vi "Get Column Info.vi"(8 "error in (no error)":errorcluster, 9 "Column Name Array":string[](array[string]), 10 "Table Name":string, 11 "Database in":refnum<class "Database.lvclass">) -> (0 "error out":errorcluster, 2 "Column Information Array":T1(array[cluster]), 3 "Database out":refnum<class "Database.lvclass">)   [LabVIEW 2020, in "Database.lvlib" / "Database.lvclass"]
uses:
  Database.lvclass
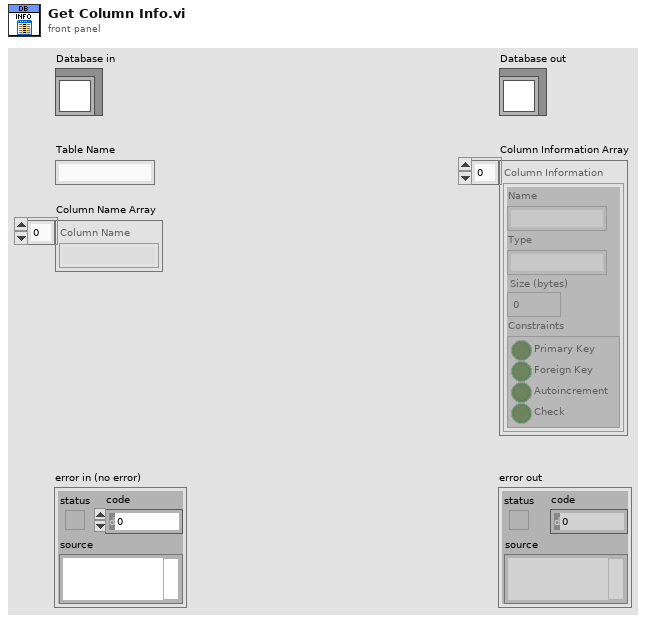
[diagram p1: front panel]
types:
  T1 = cluster{"Name":string, "Type":string, "Size (bytes)":i32, "Constraints":cluster{"Primary Key":bool, "Foreign Key":bool, "Autoincrement":bool, "Check":bool}}[]
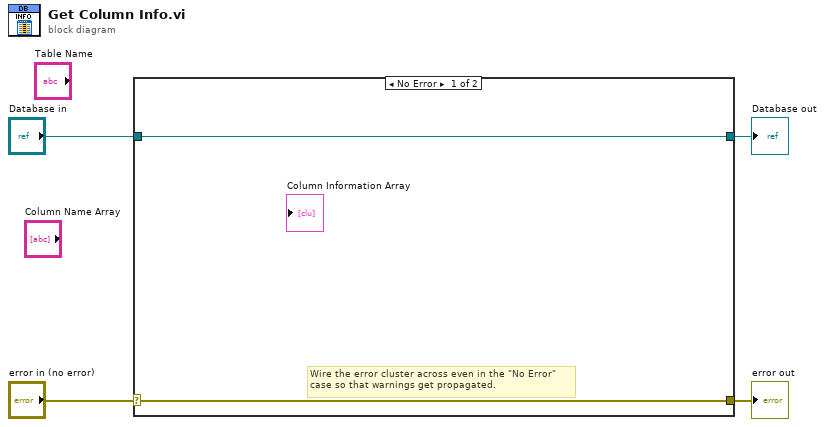
[diagram p0: block diagram]
diagram:
  n1 = case shown="No Error" "error in (no error)" {
    selector: "error in (no error)" -> [w5 w8]
    tunnel: [w5 w8] -> w3
    tunnel: [w6 w7] -> w1
    tunnel: "Database in" -> [w6 w7]
    frame No Error {
      # "Wire the error cluster across even in the \"No Error\"\ncase so that warnings get propagated."
    }
    frame Error {
    }
  }
  "error out" <- w3
  "Database out" <- w1
